vi "Divisor.vi"(8 "error in (no error)":errorcluster, 11 "Monkey in":refnum<class "Monkey.lvclass">) -> (0 "error out":errorcluster, 2 "Div Test":T1, 3 "Monkey out":refnum<class "Monkey.lvclass">)   [LabVIEW 2022 SP3, in "AoC22.lvlib" / "Monkey.lvclass"]
uses:
  Monkey.lvclass
  Monkey.lvclass/Monkey.ctl
  Worry Level.ctl
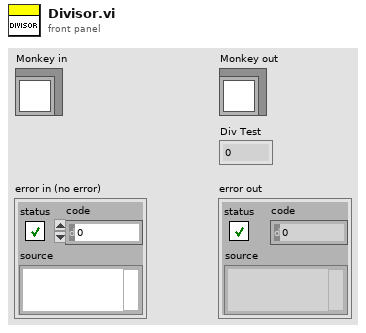
[diagram p1: front panel]
types:
  T1 = typedef "AoC22.lvlib/Monkey.lvclass/Worry Level.ctl" = u64
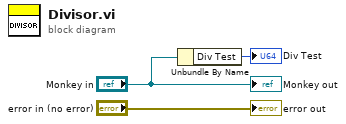
[diagram p0: block diagram]
diagram:
  n1 = Unbundle By Name("Monkey in") -> ("Div Test"=→"Div Test":T1)
  "error out" <- "error in (no error)"
  "Monkey out" <- "Monkey in"
